vi "Update Attribute By ID.vi"(8 "error in (no error)":errorcluster, 9 "Value":variant, 10 "ID":i32=-1, 11 "Attributes in":refnum<class "Attributes.lvclass">) -> (0 "error out":errorcluster, 3 "Attributes out":refnum<class "Attributes.lvclass">)   [LabVIEW 2019, in "HierDAL Library.lvlib" / "Database.lvlib" / "Repositories.lvlib" / "Attributes.lvclass"]
uses:
  Attributes.lvclass
  Attributes.lvclass/Attributes.ctl
  Database Manager Class/Database Manager.lvclass
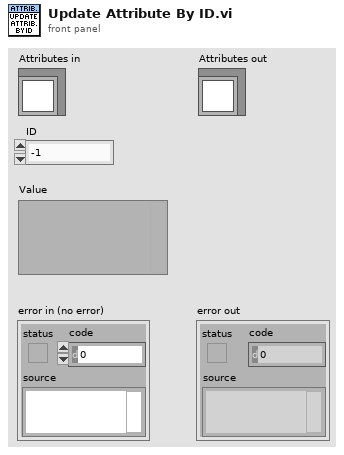
[diagram p1: front panel]
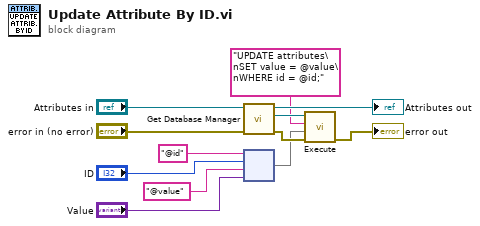
[diagram p0: block diagram]
diagram:
  n1 = call "Get Database Manager.vi"("error in (no error)"="error in (no error)", "Attributes in"="Attributes in") -> ("error out"=w8:errorcluster, "Database Manager"=w7:refnum<class "Database Manager.lvclass">, "Attributes out"=→"Attributes out":refnum<class "Attributes.lvclass">)  [unwired: 7 in]
  n2 = node("@id" ("key"), "ID", "@value" ("key"), "Value") -> (w5:map{string, variant})
  n3 = call-dynamic "Execute.vi"("error in (no error)"=w8, "Parameters"=w5, "Query"="UPDATE attributes\nSET value = @value\nWHERE id = @id;", "Database Manager in"=w7) -> ("error out"=→"error out":errorcluster)  [unwired: 6 in, 1 out]
